vi "Callback - Get Data by Name.vi"(5 "Newest Time to Plot (unix,ns)":u64, 7 "Oldest Time to Plot (unix,ns)":u64, 8 "error in (no error)":errorcluster, 10 "Name":string, 11 "BluePlotHandleDemo in":refnum<class "NIringPlotHandle.lvclass">) -> (0 "error out":errorcluster, 2 "data history":T1, 3 "BluePlotHandleDemo out":refnum<class "NIringPlotHandle.lvclass">)   [LabVIEW 2021, in "NIringPlotHandle.lvclass"]
uses:
  NIringPlotHandle.lvclass
  TypeDefs/plot datapoint.ctl
  NIringPlotHandle.lvclass/NIringPlotHandle.ctl
  Demo/SubVIs/ring buffer data.ctl
  f5e3bb7b-5070-4ac1-a4d1-7f53973bbfd5.vi
  d962ecf8-c495-4b0f-b2e1-6f431b9c5808.vi
  <userlib>/bjustice/Ring Buffer for Time Series Data Strict Accessor/Unix time epoch/Unix_Epoch_in_Labview.vi
  <userlib>/bjustice/Ring Buffer for Time Series Data Strict Accessor/SubVIs/Search for oldest time to keep.vi
  <userlib>/bjustice/Ring Buffer for Time Series Data Strict Accessor/SubVIs/Search for newest time to keep.vi
  <vilib>/National Instruments/Variant Ring Buffer/Ring Buffer.lvclass
  Demo/RocketPlotDemo.lvlib
  RocketPlot.lvlib
  <userlib>/bjustice/Ring Buffer for Time Series Data Strict Accessor/Ring Buffer Strict Accessor.lvlib
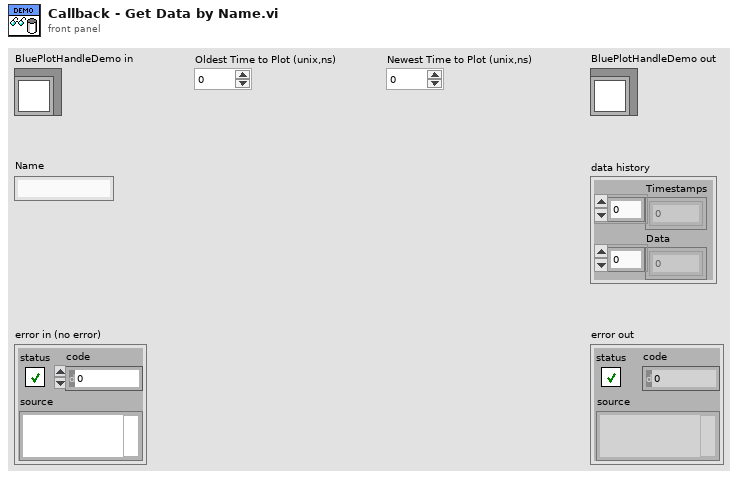
[diagram p1: front panel]
types:
  T1 = typedef "RocketPlot.lvlib/plot datapoint.ctl" = cluster{"Timestamps":u64[], "Data":dbl[]}
  T2 = typedef "RocketPlotDemo.lvlib/ring buffer data.ctl" = cluster{"timestamp":dbl, "value":dbl}
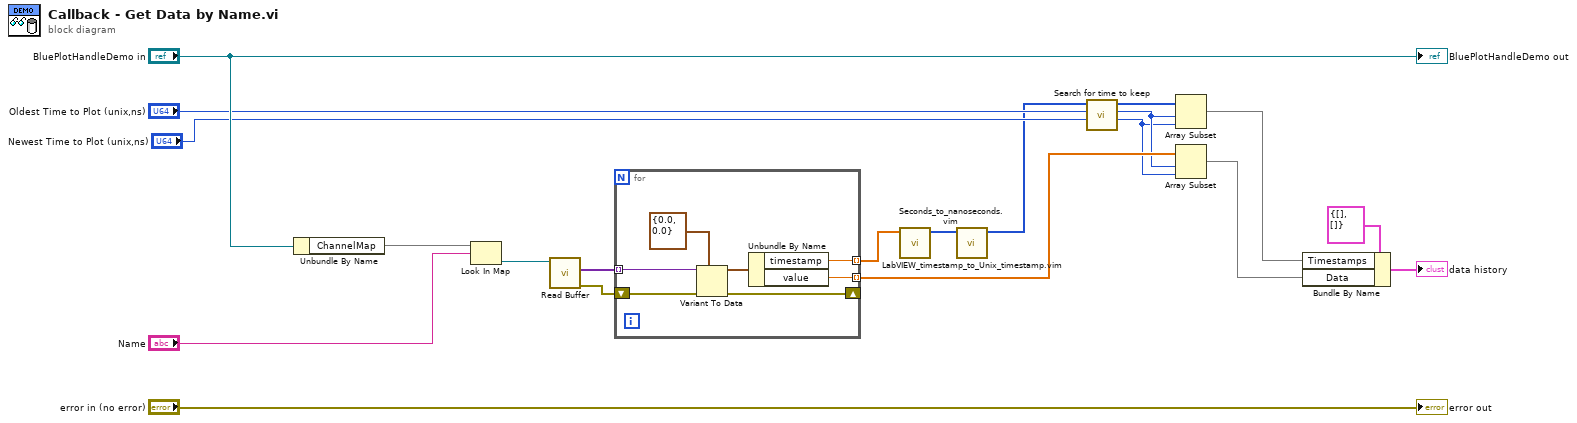
[diagram p0: block diagram]
diagram:
  n1 = Unbundle By Name("BluePlotHandleDemo in") -> ("ChannelMap"=w19:map{string, refnum<data-value>})
  n2 = Look In Map(map=w19, key="Name") -> (value=w18:refnum<data-value>)  [unwired: 1 in, 1 out]
  n3 = call <vilib>:"Read Buffer.vi"("Ring Buffer Reference"=w18) -> ("Error Out"=w14:errorcluster, "Array of Variants"=w17:variant[])  [unwired: 8 in, 1 out]
  n4 = for {
    tunnel: w17 -> [w27] mode=indexing
    tunnel: [w24] -> w2 mode=indexing
    tunnel: [w23] -> w11 mode=indexing
    shift-right: [w21] -> _
    shift-left: w14 -> [w22]
    n5 = Variant To Data(error in=w22, type=T2 {"timestamp"=0.0, "value"=0.0} ("Cluster"), Variant=w27) -> (data=w25:T2, error out=w21:errorcluster)
    n6 = Unbundle By Name(w25) -> ("timestamp"=w24:dbl, "value"=w23:dbl)
  }
  n7 = call "Seconds_to_nanoseconds.vim"("timestamp (seconds)"=w2) -> ("timestamp (nanoseconds)"=w3:u64[])  [unwired: 10 in]
  n8 = call "LabVIEW_timestamp_to_Unix_timestamp.vim"("LabVIEW timestamp (nanoseconds)"=w3) -> ("Unix timestamp (nanoseconds)"=w1:u64[])  [unwired: 10 in]
  n9 = call <userlib>:"Search for time to keep.vi"("newest time to keep"="Newest Time to Plot (unix,ns)", "oldest time to keep"="Oldest Time to Plot (unix,ns)", "timestamps (incrementing)"=w1) -> ("length"=w5:i32, "index"=w6:i32, "timestamps (dup)"=w9:u64[])  [unwired: 6 in]
  n10 = Array Subset(array=w9, index=w6, length=w5) -> (w12:u64[])
  n11 = Array Subset(array=w11, index=w6, length=w5) -> (w10:dbl[])
  n12 = Bundle By Name(cluster=T1 {"Timestamps"=[], "Data"=[]} ("data history"), "Timestamps"=w12, "Data"=w10) -> (→"data history":T1)
  "error out" <- "error in (no error)"
  "BluePlotHandleDemo out" <- "BluePlotHandleDemo in"
